vi "Auto Threshold.vi"(8 "Error In":errorcluster, 10 "Grayscale Image":T1, 11 "RGB Image":T1) -> (0 "Error Out":errorcluster, 1 "Color Plane":i32(ring)=7 items=["Red", "Green", "Blue", "Hue", "Saturation", "Luminance", "Value", "Intensity"], 2 "Inverse?":bool, 3 "Image Dst Out":T1(plugin-control))   [LabVIEW 2025]
uses:
  <vilib>/vision/Image Controls.llb/IMAQ Image.ctl
  <vilib>/vision/NI_Vision_Development_Module.lvlib
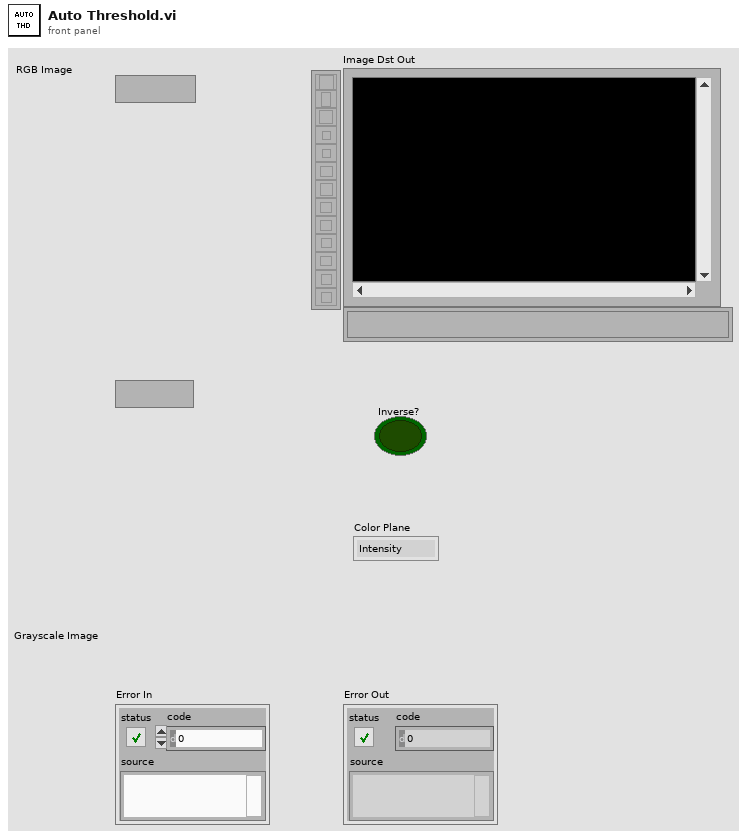
[diagram p1: front panel]
types:
  T1 = typedef "IMAQ Image.ctl" = refnum<image>
  T2 = cluster{"histogram":u32[], "Minimal Value":sgl, "Maximal Value":sgl, "Starting Value":sgl, "Interval Width":sgl, "Mean Value":sgl, "Standard  Variation":sgl, "Area (pixels)":i32}
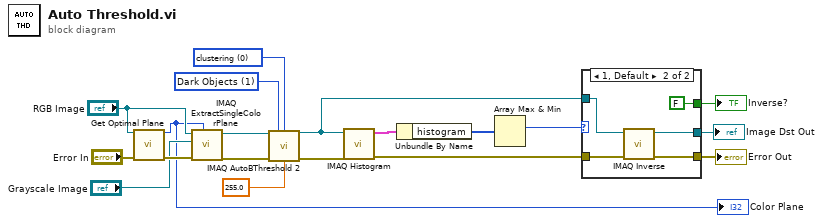
[diagram p0: block diagram]
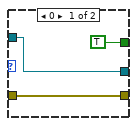
[diagram p2: hidden frame]
diagram:
  w4 = u32 1 items=["Bright Objects", "Dark Objects"] ("Look For (Bright Objects)")
  w17 = 0 items=["clustering", "entropy", "metric", "moments", "inter-class variance"] ("Method (clustering)")
  n1 = call "Get Optimal Plane.vi"("Image Src (RGB)"="RGB Image", "Error in (no error)"="Error In") -> ("Color Plane to be Extracted"=w1:i32, "Error out"=w18:errorcluster)  [unwired: 11 in, 1 out]
  "Color Plane" <- w1
  n2 = call "IMAQ ExtractSingleColorPlane"("Color Plane"=w1, "error in (no error)"=w18, "Image Dst"="Grayscale Image", "Image Src"="RGB Image") -> ("error out"=w16:errorcluster, "Image Dst Out"=w3:T1)  [unwired: 6 in]
  n3 = call "IMAQ AutoBThreshold 2"("Image Src"=w3, "Look For (Bright Objects)"=w4, "Method (clustering)"=w17, "error in (no error)"=w16, "Replace Value (1)"=sgl 255.0) -> ("Image Dst Out"=w5:T1, "error out"=w13:errorcluster)  [unwired: 8 in, 1 out]
  n4 = call "IMAQ Histogram"("error in (no error)"=w13, "Image"=w5) -> ("error out"=w10:errorcluster, "Histogram Report"=w12:T2)  [unwired: 8 in]
  n5 = Unbundle By Name(w12) -> ("histogram"=w11:u32[])
  n6 = Array Max & Min(array=w11) -> (max index (indices)=w6:i32)  [unwired: 3 out]
  n7 = case shown="1, Default" w6 {
    tunnel: w10 -> [w22 w24]
    tunnel: w5 -> [w21 w27]
    tunnel: [w22 w25] -> w8
    tunnel: [w21 w26] -> w7
    tunnel: [TRUE FALSE] -> w2
    frame 0 {
    }
    frame 1, Default {
      n8 = call "IMAQ Inverse"("error in (no error)"=w24, "Image Src"=w27) -> ("error out"=w25:errorcluster, "Image Dst Out"=w26:T1)  [unwired: 8 in]
    }
  }
  "Error Out" <- w8
  "Image Dst Out" <- w7
  "Inverse?" <- w2
